vi "main.vi"() -> ()   [LabVIEW 2020]
uses:
  status.ctl
  <vilib>/Analysis/Matrix/Datatypes/RealMatrix.ctl
  <vilib>/Analysis/3filter.llb/Savitzky-Golay Filter (DBL).vi
  <vilib>/Utility/file.llb/Read Delimited Spreadsheet (DBL).vi
  <vilib>/gmath/NumericalOptimization/Nonlinear Curve Fit LM formula string.vi
  <vilib>/gmath/NumericalOptimization/Nonlinear Curve Fit LM bound.vi
  <vilib>/Analysis/NI_AALBase.lvlib
  <vilib>/Analysis/NI_AALPro.lvlib
  <vilib>/gmath/NI_Gmath.lvlib
  <vilib>/Analysis/Matrix/NI_Matrix.lvlib
panel:
  in  "stop":bool
  in  "Tab Control":T1(tab)
  in  "file path (dialog if empty)":path
  in  "区切り文字\ndelimiter":string="\t"
  in  "y軸の列数\ncolumn num\nof y axis":i32=1
  in  "x軸の列数\ncolumn num\nof x axis":i32
  in  "LAUNCH ACTION\nACTION実行":bool
  in  "ACTION":T2
  out "XY Graph Before":T3(graph)
  out "XY Graph After":T3(graph)
  in  "CONFIRM CHANGE\n変更確定":bool
  out "XY Graph orig&baseline":T3(graph)
  in  "weight":dbl=0.0001
  in  "balance parameter":dbl=0.1
  in  "PEAKPOS ARRAY":cluster{"MIN":dbl, "MAX":dbl}[](array[cluster])
  in  "PRECISE BASELINE FIT":bool
  out "XY Graph orig&fit":T3(graph)
  in  "START FIT":bool
  in  "GAUSSIAN CLUSTER":T4
  out "resulting formula string":string
  out "R-square of fit":dbl
  in  "START CONSTRAINT FIT":bool
  out "resulting formula string constraint fit":string
  out "XY Graph orig&constraint fit":T3(graph)
  in  "Tab Control for initial params & constraint conditions":T5(tab)
  in  "GAUSSIAN CLUSTER W CONSTRAINT":T4
  in  "peakrangedata":T6
  out "R-square of constraint fit":dbl
  out "covariance":T7
  out "best fit parameters":dbl[](array[numeric])
  out "FIT RESULTS":T8(array[cluster])
  out "fit result data":cluster{"all rows":dbl[], "all rows":dbl[]}[](array[cluster])
  out "constraint fit result data":cluster{"all rows":dbl[], "all rows":dbl[]}[](array[cluster])
  # "データファイルの中に列名が入っている場合は\nあらかじめ除去してください。数字のみにしてください。\nBOM付きのデータファイルであった場合、\nBOM無しにしてください。メモ帳で確認できます。"
  # "ピークの範囲を指定してください"
  # "小さくすると、より滑らかになります"
  # "小さくすると、より指定したピーク領域を\n基線が避けるようになります"
  # "y=OFFSET+AMP*EXP(-(x-AVG)^2/(STD)^2)+..."
  # "Plot 0: sum\nLast Plot: original"
  # "OFFSET: オフセット\nAMP: 強度\nAVG: 平均\nSTD: 標準偏差"
  # "フィッテングする際の初期値を入力。"
  # "initial params: フィッテングする際の初期値を入力。"
  # "constraint conditions: フィッテングの際に変動するパラメータの可動範囲を入力。"
  # "NOTE:\n2024/2/13: added all functionalities\n2023/2/14: fixed issuses with event structure\nalso added R-square value"
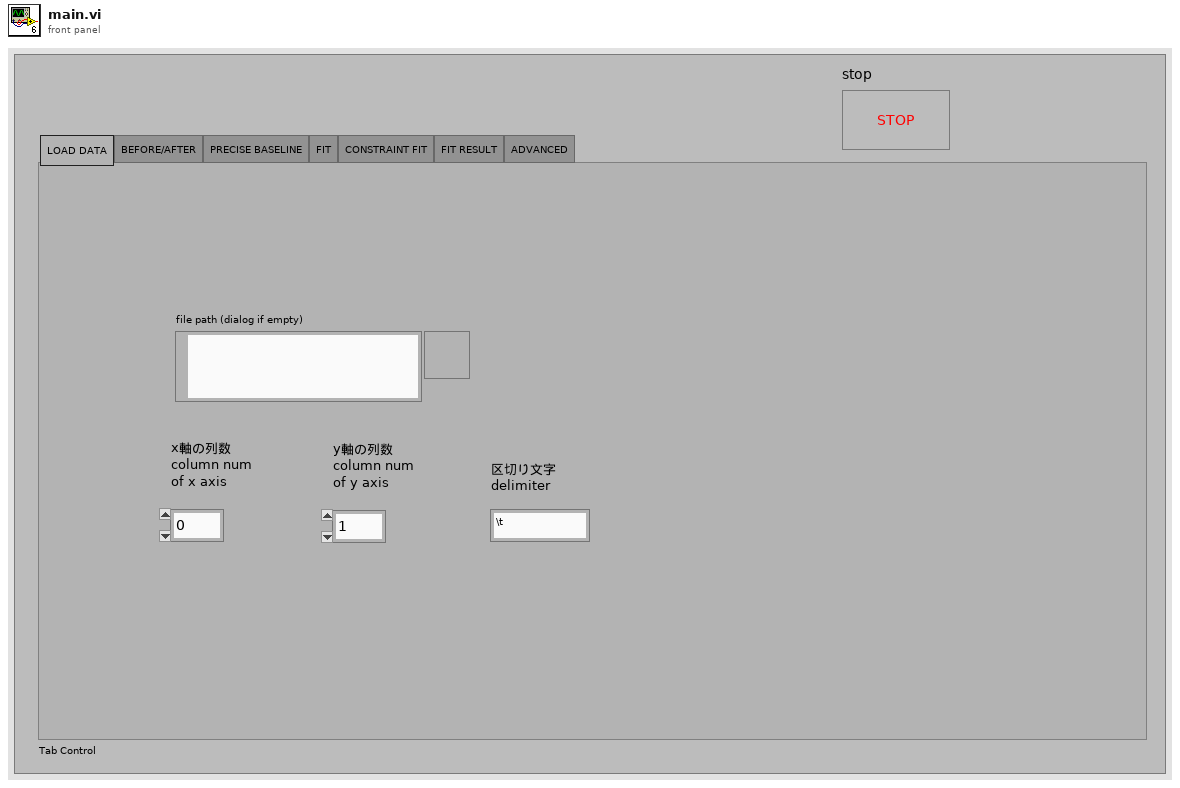
[diagram p1: front panel]
types:
  T1 = enum32{"LOAD DATA", "BEFORE/AFTER", "PRECISE BASELINE", "FIT", "CONSTRAINT FIT", "FIT RESULT", "ADVANCED"}
  T2 = typedef "status.ctl" = enum16{"INIT", "SMOOTH", "BASELINE", "FIT", "TRIM", "CONSTRAINT FIT", "PRECISE BASELINE", "CONFIRM"}
  T3 = cluster{"all rows":dbl[], "best nonlinear fit":dbl[]}[]
  T4 = cluster{"GAUSSIAN ARRAY":cluster{"AMP":dbl, "AVG":dbl, "STD":dbl}[], "OFFSET":dbl}
  T5 = enum32{"initial params", "constraint conditions"}
  T6 = cluster{"peakarray":cluster{"amprange":cluster{"min":dbl, "max":dbl}, "avgrange":cluster{"min":dbl, "max":dbl}, "stdrange":cluster{"min":dbl, "max":dbl}}[], "offsetrange":cluster{"min":dbl, "max":dbl}}
  T7 = typedef "NI_Matrix.lvlib/RealMatrix.ctl" = dbl[][]
  T8 = cluster{"AMP":dbl, "AVG":dbl, "STD":dbl, "FWHM":dbl}[]
  T9 = enum8{"Enabled", "Disabled", "Disabled and Grayed Out"}
  T10 = cluster{"all rows":dbl[], "Best Cubic Spline Fit":dbl[]}
  T11 = cluster{"all rows":dbl[], "Best Cubic Spline Fit":dbl[]}[]
  T12 = cluster{"model":string, "Parameters":string[], "x":string}
  T13 = cluster{"all rows":dbl[], "best nonlinear fit":dbl[]}
  T14 = cluster{"parameter minimum":dbl[], "parameter maximum":dbl[]}
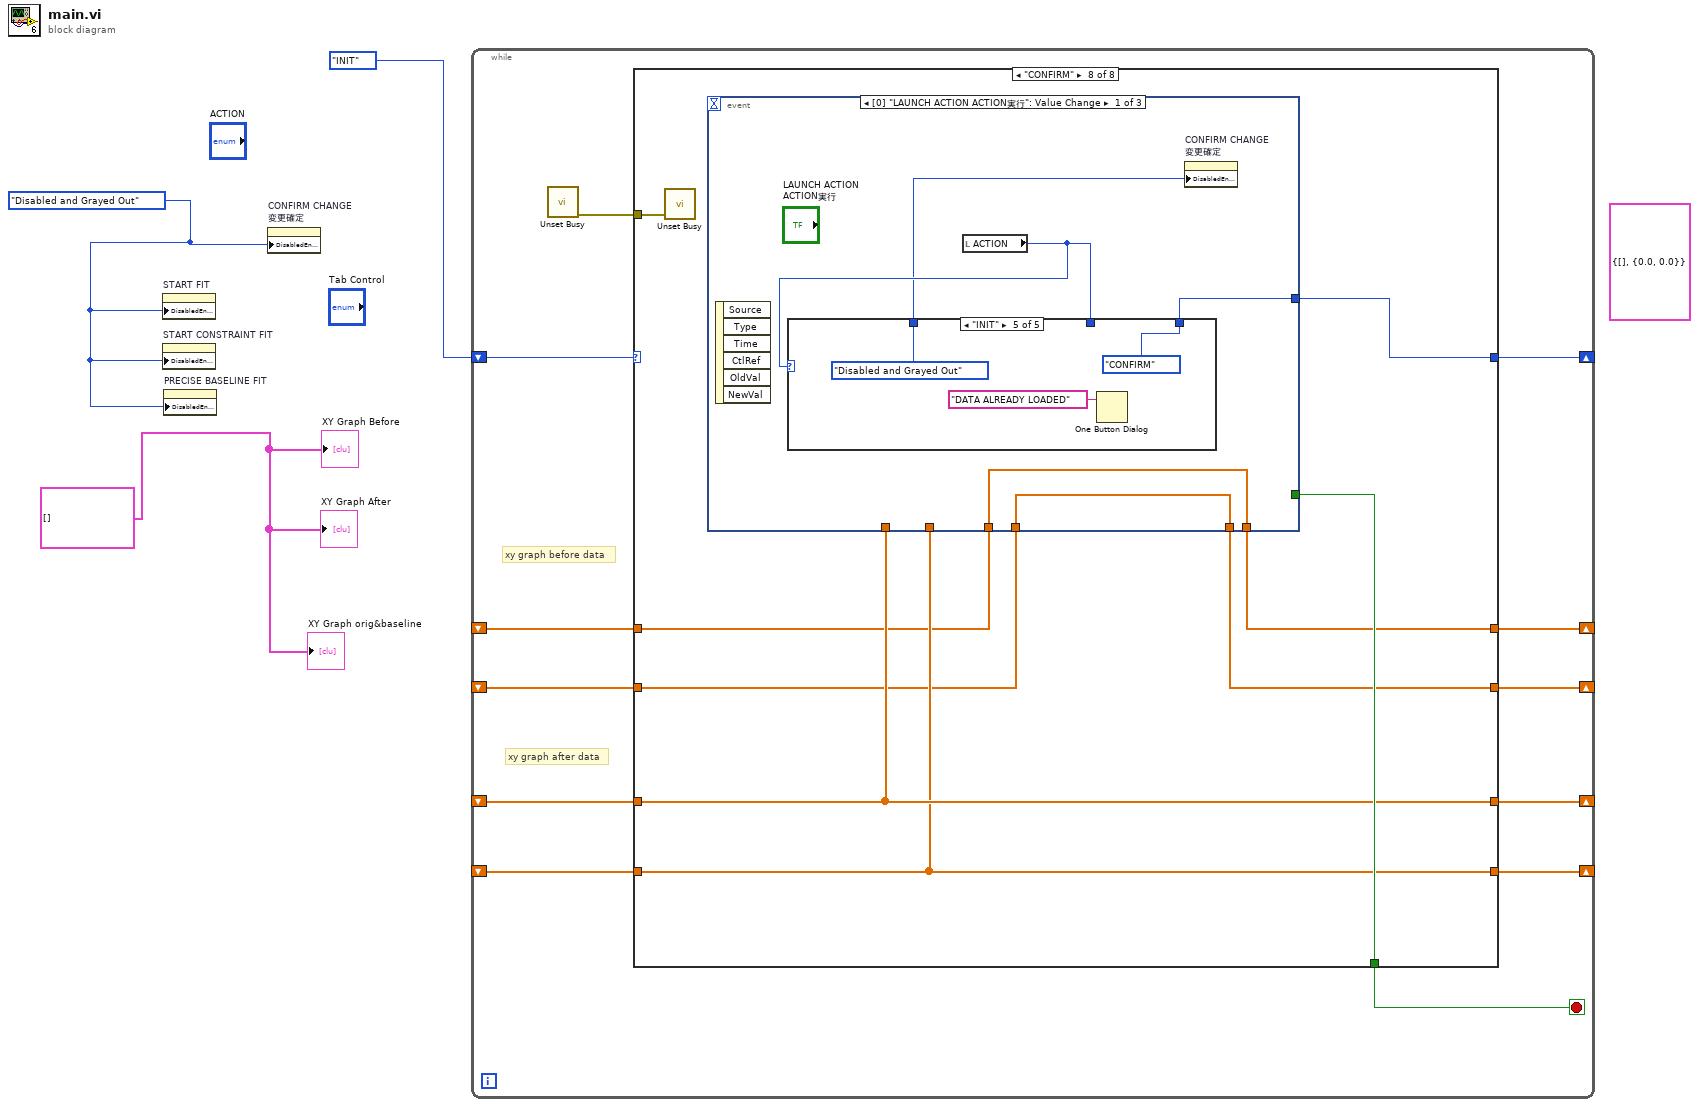
[diagram p0: block diagram]
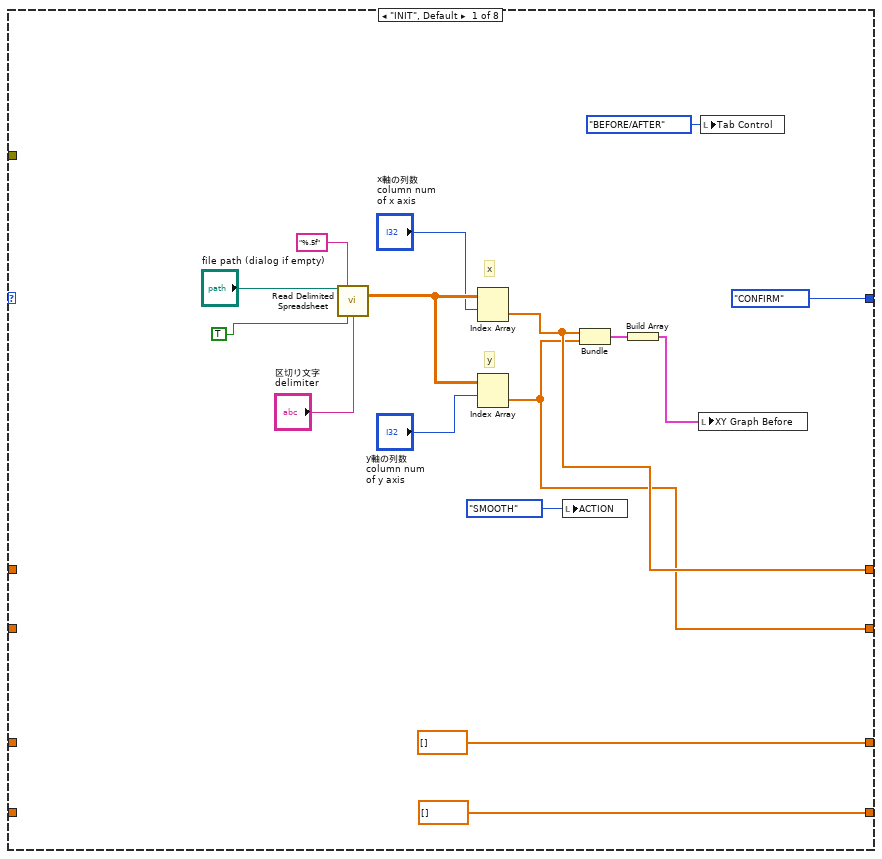
[diagram p2: hidden frame]
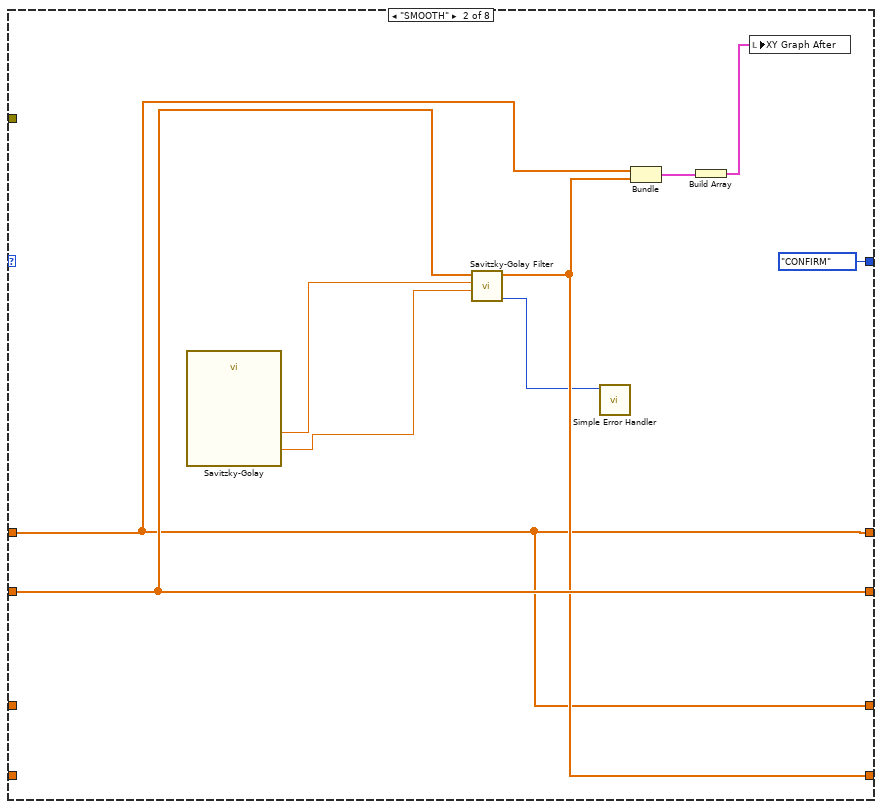
[diagram p3: hidden frame]
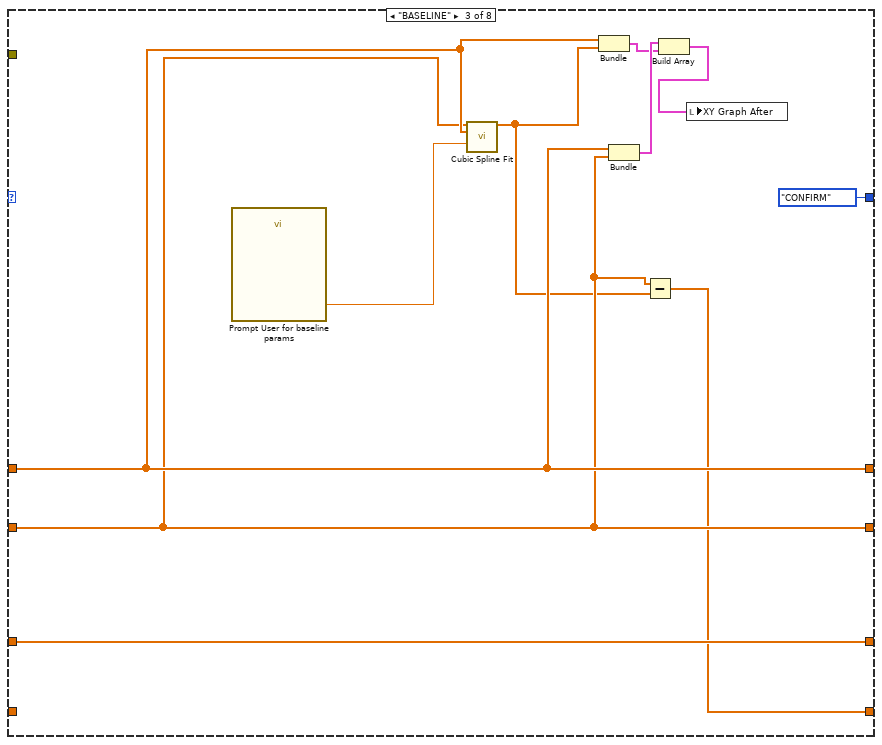
[diagram p4: hidden frame]
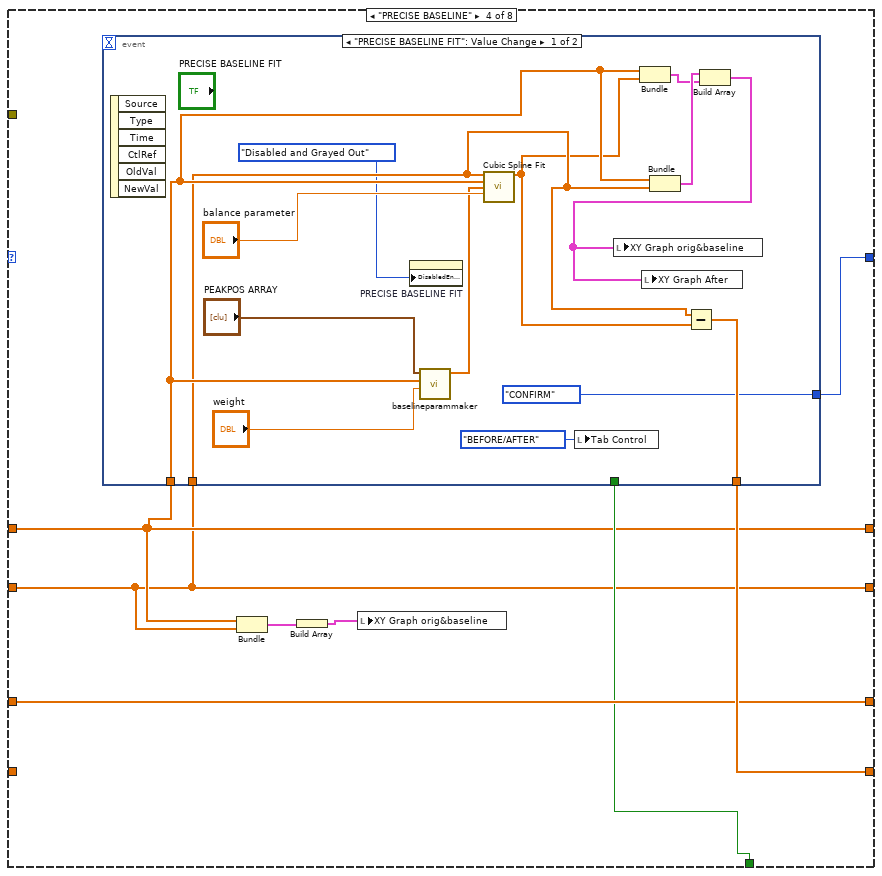
[diagram p5: hidden frame]
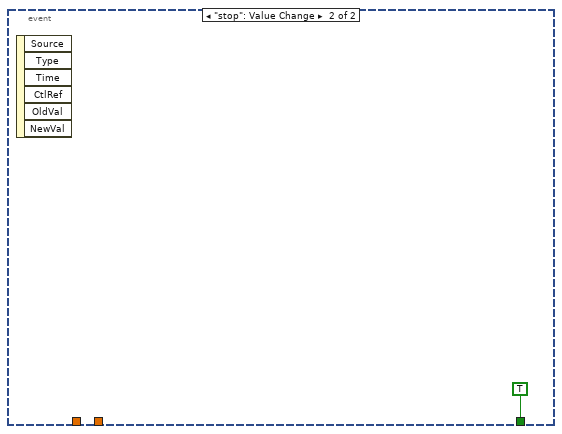
[diagram p6: hidden frame]
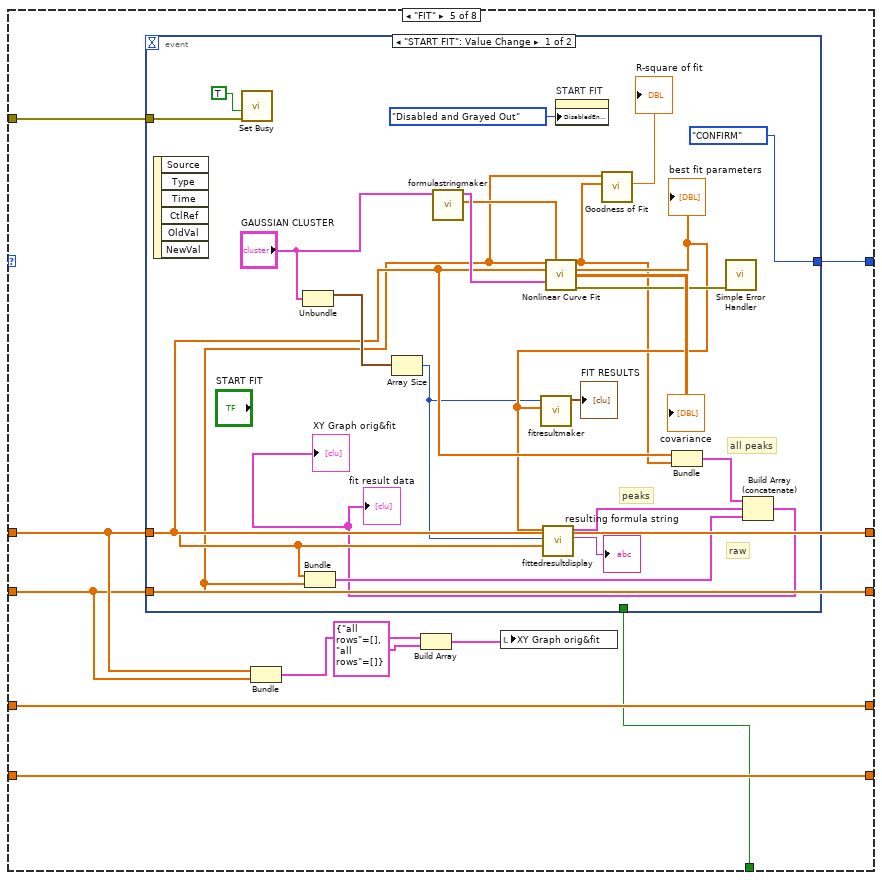
[diagram p7: hidden frame]
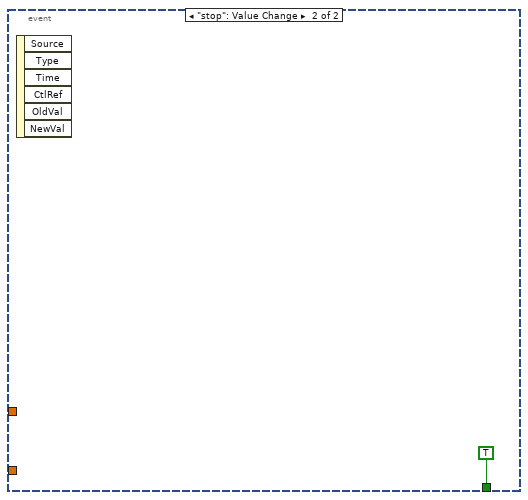
[diagram p8: hidden frame]
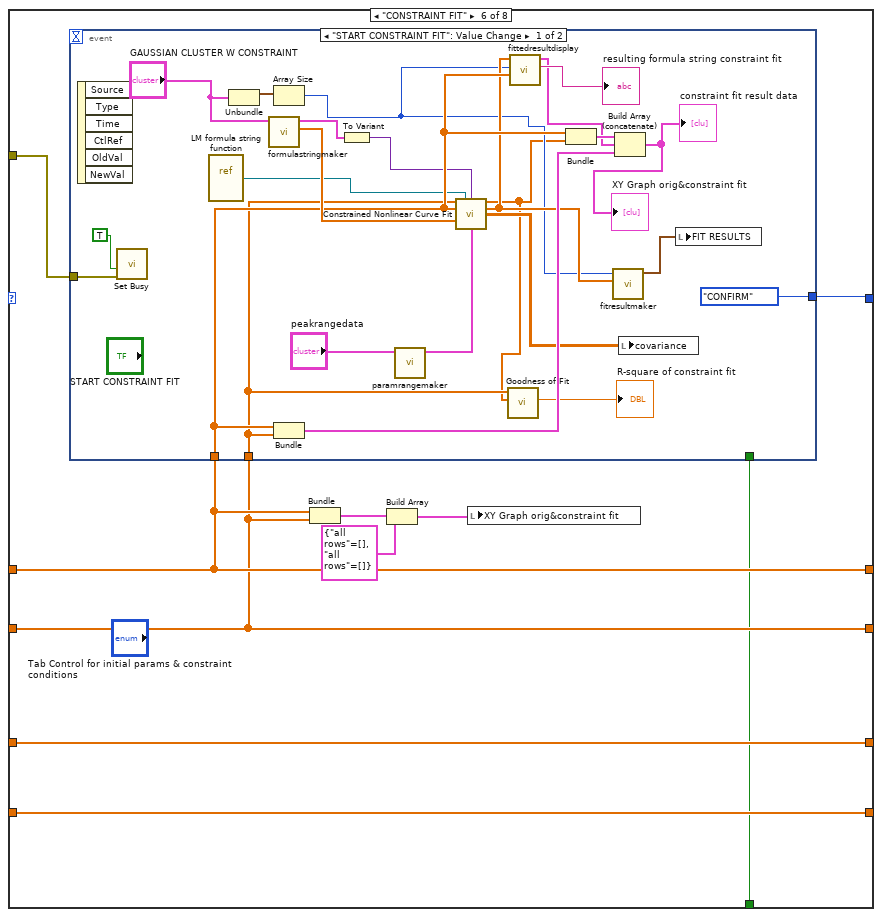
[diagram p9: hidden frame]
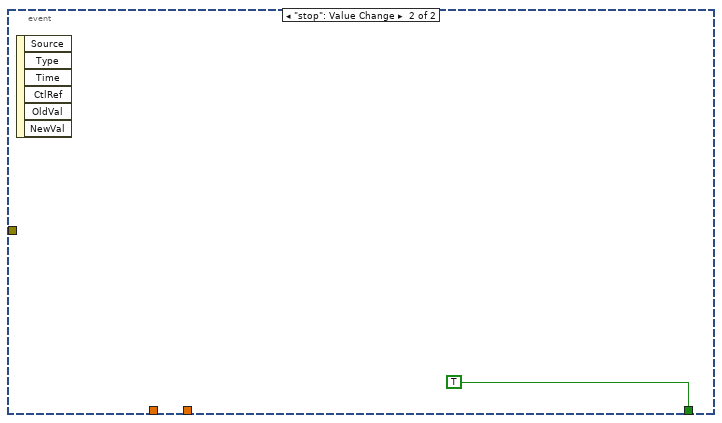
[diagram p10: hidden frame]
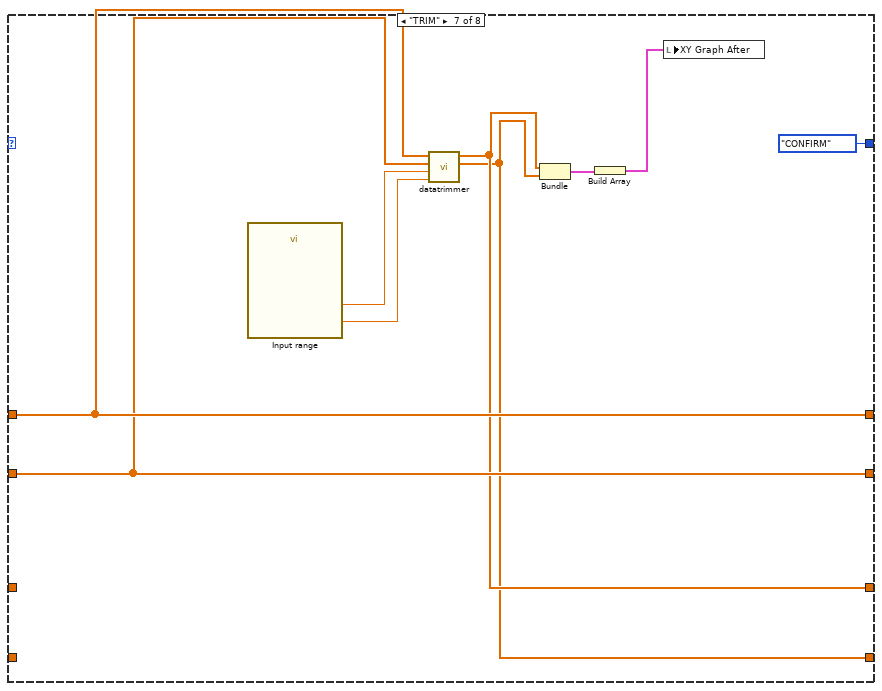
[diagram p11: hidden frame]
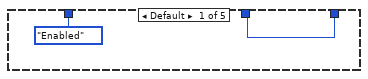
[diagram p12: hidden frame]
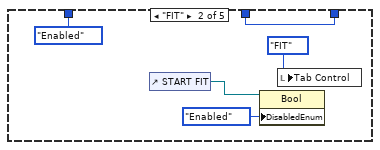
[diagram p13: hidden frame]
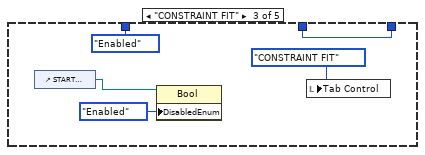
[diagram p14: hidden frame]
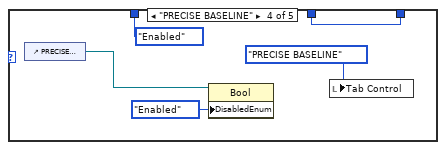
[diagram p15: hidden frame]
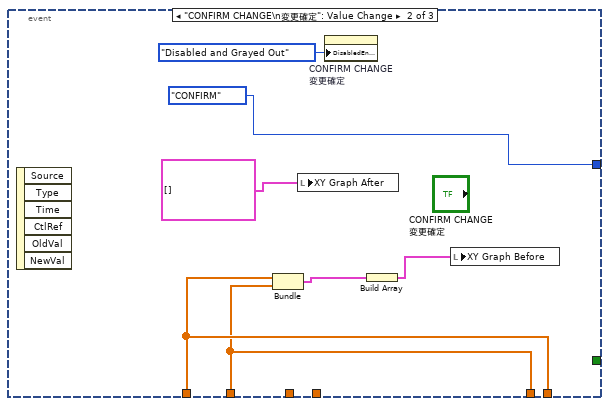
[diagram p16: hidden frame]
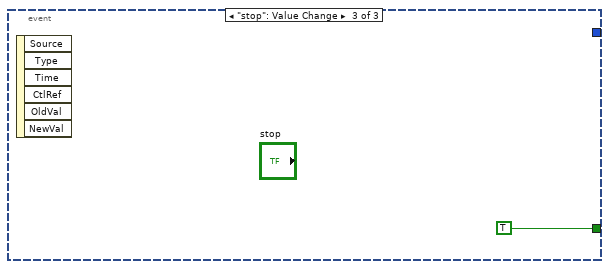
[diagram p17: hidden frame]
diagram:
  (unwired) T6 {"peakarray"=[], "offsetrange"={"min"=0.0, "max"=0.0}} ("peakrangedata")
  w1 = T9."Disabled and Grayed Out" ("Disabled")
  w2 = T3 [] ("appended array")
  n1 = property on="START FIT" class="Bool"("DisabledEnum"=w1) -> ()  [unwired: 2 in, 2 out]
  n2 = property on="START CONSTRAINT FIT" class="Bool"("DisabledEnum"=w1) -> ()  [unwired: 2 in, 2 out]
  n3 = property on="PRECISE BASELINE FIT" class="Bool"("DisabledEnum"=w1) -> ()  [unwired: 2 in, 2 out]
  n4 = property on="CONFIRM CHANGE\n変更確定" class="Bool"("DisabledEnum"=w1) -> ()  [unwired: 2 in, 2 out]
  n5 = while {
    shift-right: [w14] -> _
    shift-left: status."INIT" -> [w15]
    shift-right: [w12] -> _
    shift-left: _ -> [w10]
    shift-right: [w11] -> _
    shift-left: _ -> [w9]
    shift-right: [w8] -> _
    shift-left: _ -> [w6]
    shift-right: [w7] -> _
    shift-left: _ -> [w5]
    stop <- w13 stop-if-true
    # "xy graph after data"
    # "xy graph before data"
    n6 = call <vilib>:"Unset Busy.vi"() -> ("error out"=w4:errorcluster)  [unwired: 11 in]
    n7 = case shown="\"CONFIRM\"" w15 {
      tunnel: [status."CONFIRM" status."CONFIRM" ("NEXT") status."CONFIRM" ("NEXT") w56 w78 w116 status."CONFIRM" ("NEXT") w158] -> w14
      tunnel: [_ _ _ w55 w75 w108 _ w159] -> w13
      tunnel: [w22 w32 w46 w54 w83 w113 w147 w153] -> w12
      tunnel: [w21 w39 w43 w53 w82 w112 w146 w152] -> w11
      tunnel: w10 -> [_ w32 w46 w54 w83 w113 w147 w155]
      tunnel: w9 -> [_ w39 w43 w53 w82 w112 w146 w154]
      tunnel: [dbl[] [] ("subarray") w32 w48 w57 w77 w115 w145 w157] -> w8
      tunnel: [dbl[] [] ("subarray") w38 w41 w58 w76 w114 w144 w156] -> w7
      tunnel: w6 -> [_ _ w48 w57 w77 w115 _ w157]
      tunnel: w5 -> [_ _ _ _ w76 w114 _ w156]
      tunnel: w4 -> [_ _ _ _ w74 w107 _ w151]
      frame "INIT", Default {
        # "y"
        # "x"
        n8 = call-poly <vilib>:"Read Delimited Spreadsheet.vi"("file path (dialog if empty)"="file path (dialog if empty)", "format (%.3f)"="%.5f", "transpose? (F)"=TRUE, "delimiter (\\t)"="区切り文字\ndelimiter") -> ("all rows"=w30:dbl[][])  [unwired: 6 in, 5 out]
        n9 = Index Array(array=w30, index (row)="x軸の列数\ncolumn num\nof x axis") -> (element=w22:dbl[])  [unwired: 1 in]
        n10 = Index Array(array=w30, index (row)="y軸の列数\ncolumn num\nof y axis") -> (element=w21:dbl[])  [unwired: 1 in]
        n11 = local write "ACTION"(status."SMOOTH" ("NEXT MODE")) -> ()
        n12 = Bundle("all rows"=w22, "all rows"=w21) -> (w18:cluster{"all rows":dbl[], "all rows":dbl[]})  [unwired: 1 in]
        n13 = Build Array(w18) -> (w17:cluster{"all rows":dbl[], "all rows":dbl[]}[])
        n14 = local write "XY Graph Before"(w17) -> ()
        n15 = local write "Tab Control"(T1."BEFORE/AFTER" ("Tab Control")) -> ()
      }
      frame "SMOOTH" {
        n16 = call "Savitzky-Golay"() -> ("polyorder"=w36:dbl, "window length"=w37:dbl)  [unwired: 16 in, 2 out]
        n17 = call-poly <vilib>:"Savitzky-Golay Filter.vi"("polynomial order"=w36, "side points"=w37, "X"=w39) -> ("error"=w35:i32, "Filtered X"=w38:dbl[])  [unwired: 7 in]
        n18 = call <vilib>:"Simple Error Handler.vi"("error code (no error:0)"=w35) -> ()  [unwired: 4 in, 5 out]
        n19 = Bundle("all rows"=w32, "Filtered X"=w38) -> (w34:cluster{"all rows":dbl[], "Filtered X":dbl[]})  [unwired: 1 in]
        n20 = Build Array(w34) -> (w33:cluster{"all rows":dbl[], "Filtered X":dbl[]}[])
        n21 = local write "XY Graph After"(w33) -> ()
      }
      frame "BASELINE" {
        n22 = call "Prompt User for baseline params"() -> ("balnce parameter"=w49:dbl)  [unwired: 17 in, 2 out]
        n23 = call <vilib>:"Cubic Spline Fit.vi"("Y"=w43, "X"=w46, "balance parameter"=w49) -> ("Best Cubic Spline Fit"=w42:dbl[])  [unwired: 11 in, 1 out]
        n24 = Bundle("all rows"=w46, "Best Cubic Spline Fit"=w42) -> (w44:T10)  [unwired: 1 in]
        n25 = Bundle("all rows"=w46, "all rows"=w43) -> (w45:cluster{"all rows":dbl[], "all rows":dbl[]})  [unwired: 1 in]
        n26 = Subtract(x=w43, y=w42) -> (x-y=w41:dbl[])
        n27 = Build Array(w45, w44) -> (w47:T11)
        n28 = local write "XY Graph After"(w47) -> ()
      }
      frame "PRECISE BASELINE" {
        n29 = event shown="[0] \"PRECISE BASELINE FIT\": Value Change" {
          selector: _ -> [_ _]
          dyn-events: _ -> [_ _]
          timeout: _ -> [_ _]
          tunnel: w54 -> [w66 _]
          tunnel: w53 -> [w65 _]
          tunnel: [w63 _] -> w58
          tunnel: [status."CONFIRM" ("NEXT MODE") _] -> w56
          tunnel: [_ TRUE] -> w55
          event "PRECISE BASELINE FIT": Value Change {
            n30 = event-data() -> ()  [unwired: 1 in, 6 out]
            n31 = property on="PRECISE BASELINE FIT" class="Bool"("DisabledEnum"=T9."Disabled and Grayed Out" ("Disabled")) -> ()  [unwired: 2 in, 2 out]
            n32 = call "baselineparammaker.vi"("weight <1"="weight", "x"=w66, "PEAKPOS ARRAY"="PEAKPOS ARRAY") -> ("weight array"=w69:dbl[])  [unwired: 8 in]
            n33 = call <vilib>:"Cubic Spline Fit.vi"("Y"=w65, "X"=w66, "Weight"=w69, "balance parameter"="balance parameter") -> ("Best Cubic Spline Fit"=w64:dbl[])  [unwired: 10 in, 1 out]
            n34 = local write "Tab Control"(T1."BEFORE/AFTER" ("Tab Control")) -> ()
            n35 = Bundle("all rows"=w66, "Best Cubic Spline Fit"=w64) -> (w67:T10)  [unwired: 1 in]
            n36 = Bundle("all rows"=w66, "all rows"=w65) -> (w68:cluster{"all rows":dbl[], "all rows":dbl[]})  [unwired: 1 in]
            n37 = Subtract(x=w65, y=w64) -> (x-y=w63:dbl[])
            n38 = Build Array(w68, w67) -> (w61:T11)
            n39 = local write "XY Graph orig&baseline"(w61) -> ()
            n40 = local write "XY Graph After"(w61) -> ()
          }
          event "stop": Value Change {
            n41 = event-data() -> ()  [unwired: 1 in, 6 out]
          }
        }
        n42 = Bundle("all rows"=w54, "all rows"=w53) -> (w51:cluster{"all rows":dbl[], "all rows":dbl[]})  [unwired: 1 in]
        n43 = Build Array(w51) -> (w52:cluster{"all rows":dbl[], "all rows":dbl[]}[])
        n44 = local write "XY Graph orig&baseline"(w52) -> ()
      }
      frame "FIT" {
        n45 = event shown="[0] \"START FIT\": Value Change" {
          selector: _ -> [_ _]
          dyn-events: _ -> [_ _]
          timeout: _ -> [_ _]
          tunnel: w83 -> [w96 _]
          tunnel: w82 -> [w86 _]
          tunnel: [status."CONFIRM" ("NEXT") _] -> w78
          tunnel: [_ TRUE] -> w75
          tunnel: w74 -> [w89 _]
          event "START FIT": Value Change {
            # "raw"
            # "all peaks"
            # "peaks"
            n46 = event-data() -> ()  [unwired: 1 in, 6 out]
            n47 = call <vilib>:"Set Busy.vi"("error in (no error)"=w89, "disable click? (T)"=TRUE) -> ()  [unwired: 8 in, 2 out]
            n48 = Unbundle("GAUSSIAN CLUSTER") -> ("GAUSSIAN ARRAY"=w99:cluster{"AMP":dbl, "AVG":dbl, "STD":dbl}[])  [unwired: 1 out]
            n49 = Bundle("all rows"=w96, "all rows"=w86) -> (w95:cluster{"all rows":dbl[], "all rows":dbl[]})  [unwired: 1 in]
            n50 = Array Size(array=w99) -> (size(s)=w92:i32)
            n51 = call "formulastringmaker.vi"("GAUSSIAN CLUSTER"="GAUSSIAN CLUSTER") -> ("initial parameters"=w104:dbl[], "output model"=w105:T12)  [unwired: 9 in]
            n52 = call-poly <vilib>:"Nonlinear Curve Fit.vi"("Y"=w86, "initial parameters"=w104, "X"=w96, "model description"=w105) -> ("best nonlinear fit"=w85:dbl[], "best fit parameters"=w93:dbl[], "covariance"=→"covariance":T7, "error out"=w101:errorcluster)  [unwired: 7 in, 1 out]
            "best fit parameters" <- w93
            n53 = call "fitresultmaker.vi"("best fit parameter"=w93, "num of gaussian peaks"=w92) -> ("FIT RESULTS"=→"FIT RESULTS":T8)  [unwired: 9 in]
            n54 = call "fittedresultdisplay.vi"("x"=w96, "num of gaussian peaks"=w92, "best fit parameters"=w93) -> ("resulting formula string"=→"resulting formula string":string, "all gaussian points"=w97:T3)  [unwired: 7 in]
            n55 = property on="START FIT" class="Bool"("DisabledEnum"=T9."Disabled and Grayed Out" ("Disabled")) -> ()  [unwired: 2 in, 2 out]
            n56 = call <vilib>:"Goodness of Fit.vi"("Best Fit"=w85, "Y"=w86) -> ("R-square"=→"R-square of fit":dbl)  [unwired: 6 in, 3 out]
            n57 = Bundle("all rows"=w96, "best nonlinear fit"=w85) -> (w98:T13)  [unwired: 1 in]
            n58 = call <vilib>:"Simple Error Handler.vi"("error in (no error)"=w101) -> ()  [unwired: 4 in, 5 out]
            n59 = Build Array (concatenate)(w98, w97, w95) -> (→"XY Graph orig&fit" →"fit result data":cluster{"all rows":dbl[], "all rows":dbl[]}[])
          }
          event "stop": Value Change {
            n60 = event-data() -> ()  [unwired: 1 in, 6 out]
          }
        }
        n61 = Bundle("all rows"=w83, "all rows"=w82) -> (w81:cluster{"all rows":dbl[], "all rows":dbl[]})  [unwired: 1 in]
        n62 = Build Array(w81, cluster{"all rows":dbl[], "all rows":dbl[]} {"all rows"=[], "all rows"=[]} ("element")) -> (w80:cluster{"all rows":dbl[], "all rows":dbl[]}[])
        n63 = local write "XY Graph orig&fit"(w80) -> ()
      }
      frame "CONSTRAINT FIT" {
        n64 = event shown="[0] \"START CONSTRAINT FIT\": Value Change" {
          selector: _ -> [_ _]
          dyn-events: _ -> [_ _]
          timeout: _ -> [_ _]
          tunnel: w113 -> [w133 _]
          tunnel: w112 -> [w119 _]
          tunnel: [status."CONFIRM" ("NEXT MODE") _] -> w116
          tunnel: [_ TRUE] -> w108
          tunnel: w107 -> [w123 _]
          event "START CONSTRAINT FIT": Value Change {
            n65 = event-data() -> ()  [unwired: 1 in, 6 out]
            n66 = call <vilib>:"Set Busy.vi"("error in (no error)"=w123, "disable click? (T)"=TRUE) -> ()  [unwired: 8 in, 2 out]
            n67 = vi-ref <vilib>:"LM formula string function.vi"() -> ("vi reference"=w125:refnum<vi>)
            n68 = Unbundle("GAUSSIAN CLUSTER W CONSTRAINT") -> ("GAUSSIAN ARRAY"=w137:cluster{"AMP":dbl, "AVG":dbl, "STD":dbl}[])  [unwired: 1 out]
            n69 = call "formulastringmaker.vi"("GAUSSIAN CLUSTER"="GAUSSIAN CLUSTER W CONSTRAINT") -> ("initial parameters"=w139:dbl[], "output model"=w140:T12)  [unwired: 9 in]
            n70 = Array Size(array=w137) -> (size(s)=w128:i32)
            n71 = Bundle("all rows"=w133, "all rows"=w119) -> (w132:cluster{"all rows":dbl[], "all rows":dbl[]})  [unwired: 1 in]
            n72 = To Variant(anything=w140) -> (Variant=w124:variant)
            n73 = call "paramrangemaker.vi"("peakrangedata"="peakrangedata") -> ("parameter bounds out"=w121:T14)  [unwired: 10 in]
            n74 = call-poly <vilib>:"Constrained Nonlinear Curve Fit.vi"("Y"=w119, "f(x,a)"=w125, "data"=w124, "X"=w133, "initial parameters"=w139, "parameter bounds"=w121) -> ("best nonlinear fit"=w118:dbl[], "best fit parameters"=w129:dbl[], "covariance"=w126:T7)  [unwired: 4 in, 3 out]
            n75 = call <vilib>:"Goodness of Fit.vi"("Best Fit"=w118, "Y"=w119) -> ("R-square"=→"R-square of constraint fit":dbl)  [unwired: 6 in, 3 out]
            n76 = call "fittedresultdisplay.vi"("x"=w133, "num of gaussian peaks"=w128, "best fit parameters"=w129) -> ("resulting formula string"=→"resulting formula string constraint fit":string, "all gaussian points"=w134:T3)  [unwired: 7 in]
            n77 = Bundle("all rows"=w133, "best nonlinear fit"=w118) -> (w135:T13)  [unwired: 1 in]
            n78 = call "fitresultmaker.vi"("best fit parameter"=w129, "num of gaussian peaks"=w128) -> ("FIT RESULTS"=w127:T8)  [unwired: 9 in]
            n79 = Build Array (concatenate)(w135, w134, w132) -> (→"XY Graph orig&constraint fit" →"constraint fit result data":cluster{"all rows":dbl[], "all rows":dbl[]}[])
            n80 = local write "covariance"(w126) -> ()
            n81 = local write "FIT RESULTS"(w127) -> ()
          }
          event "stop": Value Change {
            n82 = event-data() -> ()  [unwired: 1 in, 6 out]
          }
        }
        n83 = Bundle("all rows"=w113, "all rows"=w112) -> (w110:cluster{"all rows":dbl[], "all rows":dbl[]})  [unwired: 1 in]
        n84 = Build Array(w110, cluster{"all rows":dbl[], "all rows":dbl[]} {"all rows"=[], "all rows"=[]} ("element")) -> (w111:cluster{"all rows":dbl[], "all rows":dbl[]}[])
        n85 = local write "XY Graph orig&constraint fit"(w111) -> ()
      }
      frame "TRIM" {
        n86 = call "Input range"() -> ("max x"=w148:dbl, "min x"=w149:dbl)  [unwired: 16 in, 2 out]
        n87 = call "datatrimmer.vi"("max x"=w148, "min x"=w149, "y"=w146, "x"=w147) -> ("trimmed y"=w144:dbl[], "trimmed x"=w145:dbl[])  [unwired: 6 in]
        n88 = Bundle("trimmed x"=w145, "trimmed y"=w144) -> (w143:cluster{"trimmed x":dbl[], "trimmed y":dbl[]})  [unwired: 1 in]
        n89 = Build Array(w143) -> (w142:cluster{"trimmed x":dbl[], "trimmed y":dbl[]}[])
        n90 = local write "XY Graph After"(w142) -> ()
      }
      frame "CONFIRM" {
        n91 = call <vilib>:"Unset Busy.vi"("error in (no error)"=w151) -> ()  [unwired: 10 in, 1 out]
        n92 = event shown="[0] \"LAUNCH ACTION ACTION実行\": Value Change" {
          selector: _ -> [_ _ _]
          dyn-events: _ -> [_ _ _]
          timeout: _ -> [_ _ _]
          tunnel: [_ _ TRUE] -> w159
          tunnel: [w162 status."CONFIRM" ("NEXT MODE") _] -> w158
          tunnel: w157 -> [_ w190 _]
          tunnel: w156 -> [_ w189 _]
          tunnel: w155 -> [w164 _ _]
          tunnel: w154 -> [w163 _ _]
          tunnel: [w164 w190 _] -> w153
          tunnel: [w163 w189 _] -> w152
          event "LAUNCH ACTION\nACTION実行": Value Change {
            n93 = event-data() -> ()  [unwired: 1 in, 6 out]
            n94 = local read "ACTION"() -> (w161:T2)
            n95 = case shown="\"INIT\"" w161 {
              tunnel: [w166 w168 w173 w178 status."CONFIRM" ("ACTION")] -> w162
              tunnel: w161 -> [w166 w168 w173 w178 _]
              tunnel: [T9."Enabled" ("Disabled") T9."Enabled" ("Disabled") T9."Enabled" ("Disabled") T9."Enabled" ("Disabled") T9."Disabled and Grayed Out" ("Disabled")] -> w160
              frame Default {
              }
              frame "FIT" {
                n96 = control-ref of="START FIT"() -> (w170:refnum<vi>)
                n97 = property class="Bool"(reference=w170, "DisabledEnum"=T9."Enabled" ("Disabled")) -> ()  [unwired: 1 in, 2 out]
                n98 = local write "Tab Control"(T1."FIT" ("Tab Control")) -> ()
              }
              frame "CONSTRAINT FIT" {
                n99 = control-ref of="START CONSTRAINT FIT"() -> (w175:refnum<vi>)
                n100 = property class="Bool"(reference=w175, "DisabledEnum"=T9."Enabled" ("Disabled")) -> ()  [unwired: 1 in, 2 out]
                n101 = local write "Tab Control"(T1."CONSTRAINT FIT" ("Tab Control")) -> ()
              }
              frame "PRECISE BASELINE" {
                n102 = control-ref of="PRECISE BASELINE FIT"() -> (w180:refnum<vi>)
                n103 = property class="Bool"(reference=w180, "DisabledEnum"=T9."Enabled" ("Disabled")) -> ()  [unwired: 1 in, 2 out]
                n104 = local write "Tab Control"(T1."PRECISE BASELINE" ("Tab Control")) -> ()
              }
              frame "INIT" {
                n105 = One Button Dialog(message="DATA ALREADY LOADED") -> ()  [unwired: 1 in, 1 out]
              }
            }
            n106 = property on="CONFIRM CHANGE\n変更確定" class="Bool"("DisabledEnum"=w160) -> ()  [unwired: 2 in, 2 out]
          }
          event "CONFIRM CHANGE\n変更確定": Value Change {
            n107 = event-data() -> ()  [unwired: 1 in, 6 out]
            n108 = Bundle("trimmed x"=w190, "trimmed y"=w189) -> (w188:cluster{"trimmed x":dbl[], "trimmed y":dbl[]})  [unwired: 1 in]
            n109 = local write "XY Graph After"(T3 [] ("XY Graph After")) -> ()
            n110 = property on="CONFIRM CHANGE\n変更確定" class="Bool"("DisabledEnum"=T9."Disabled and Grayed Out" ("Disabled")) -> ()  [unwired: 2 in, 2 out]
            n111 = Build Array(w188) -> (w186:cluster{"trimmed x":dbl[], "trimmed y":dbl[]}[])
            n112 = local write "XY Graph Before"(w186) -> ()
          }
          event "stop": Value Change {
            n113 = event-data() -> ()  [unwired: 1 in, 6 out]
          }
        }
      }
    }
  }
  "XY Graph Before" <- w2
  "XY Graph After" <- w2
  "XY Graph orig&baseline" <- w2
